vi "Reset all hightlights.vi"(8 "error in (no error)":errorcluster, 11 "Display State In in":T1={"logTable"=refnum, "max items"=500, "displaydata"=[], "data"=[], "Auto Scroll"=TRUE, "current item"=500, "col headers"=[], "Add to Top"=FALSE, "Auto resize"=TRUE, "col size"=[], "filters"=[], "color cells"=[]}) -> (0 "error out":errorcluster, 3 "Display State In out":T1={"logTable"=refnum, "max items"=500, "displaydata"=[], "data"=[], "Auto Scroll"=TRUE, "current item"=500, "col headers"=[], "Add to Top"=FALSE, "Auto resize"=TRUE, "col size"=[], "filters"=[], "color cells"=[]})   [LabVIEW 2013, in "UI-DisplayTable(dev).xctl"]
uses:
  UI-DisplayTable(dev).xctl
  State.ctl
  DEF-Filter.ctl
  <vilib>/Utility/miscctls.llb/LVRowAndColumnTypeDef.ctl
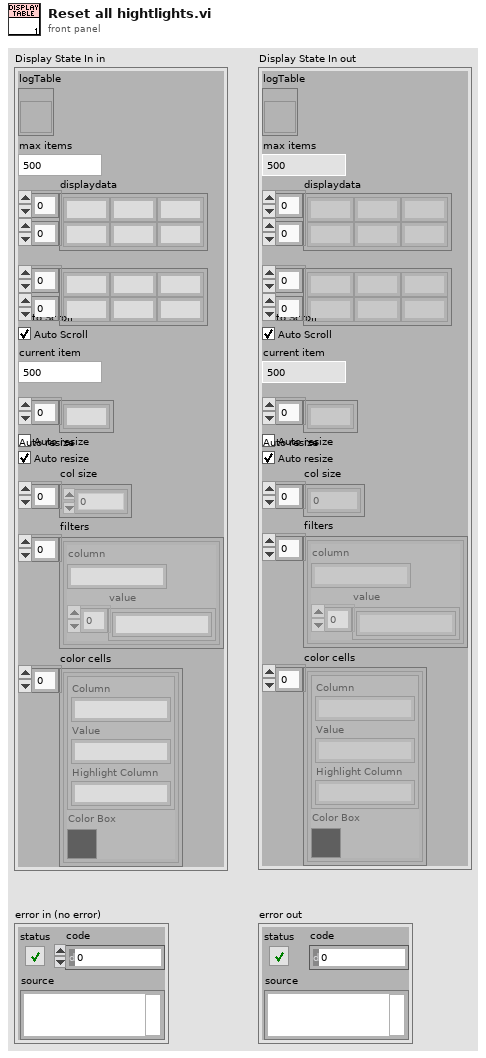
[diagram p1: front panel]
types:
  T1 = typedef "UI-DisplayTable(dev).xctl/State.ctl" = cluster{"logTable":refnum<vi>, "max items":i32, "displaydata":string[][], "data":string[][], "Auto Scroll":bool, "current item":i32, "col headers":string[], "Add to Top":bool, "Auto resize":bool, "col size":i32[], "filters":T2[], "color cells":cluster{"color cell":cluster{"Column":string, "Value":string, "Highlight Column":string}, "Color Box":u32}[]}
  T2 = typedef "UI-DisplayTable(dev).xctl/DEF-Filter.ctl" = cluster{"column":string, "value":string[]}
  T3 = typedef "LVRowAndColumnTypeDef.ctl" = cluster{"Row":i32, "Column":i32}
  T4 = cluster{"color cell":cluster{"Column":string, "Value":string, "Highlight Column":string}, "Color Box":u32}[]
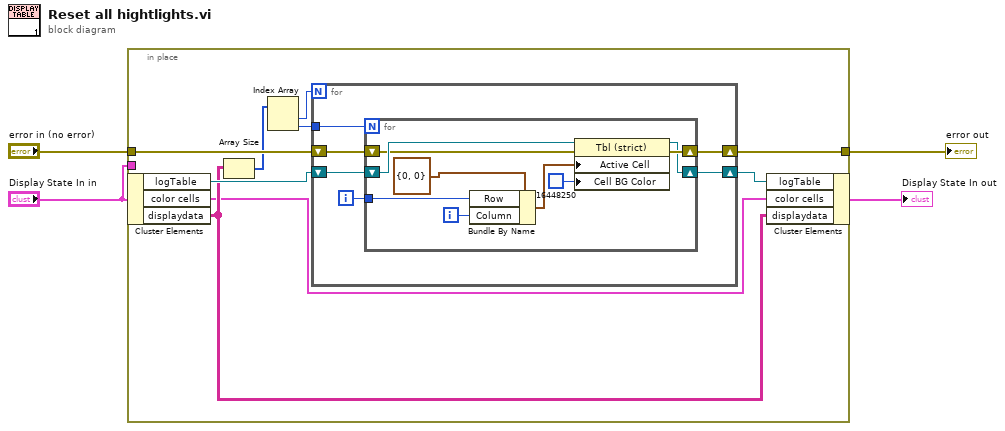
[diagram p0: block diagram]
diagram:
  n1 = in-place {
    in-place-border: "Display State In in" -> [_]
    in-place-border: "error in (no error)" -> [w13]
    in-place-border: [w12] -> w2
    n2 = in-place-cluster #1("Display State In in") -> ("logTable"=w11:refnum<vi>, "color cells"=w5:T4, "displaydata"=w9:string[][])
    n3 = Array Size(array=w9) -> (size(s)=w8:i32[])
    n4 = Index Array(array=w8) -> (element #1=w7:i32, element #2=w6:i32)  [unwired: 2 in]
    n5 = for {
      N: w7 -> [_]
      shift-right: [w17] -> w12
      shift-left: w13 -> [w18]
      shift-right: [w16] -> w10
      shift-left: w11 -> [w19]
      tunnel: w6 -> [w15]
      i -> [w14]
      n6 = for {
        N: w15 -> [_]
        shift-right: [w22] -> w16
        shift-left: w19 -> [w28]
        shift-right: [w25] -> w17
        shift-left: w18 -> [w26]
        tunnel: w14 -> [w21]
        i -> [w20]
        n7 = Bundle By Name(cluster=T3 {"Row"=0, "Column"=0} ("Active Cell:Active Cell"), "Row"=w21, "Column"=w20) -> (w23:T3)
        n8 = property class="Tbl (strict)"(reference=w28, error in=w26, "Active Cell"=w23, "Cell BG Color"=u32 16448250 ("Active Cell:Cell Background Color")) -> (reference out=w22:refnum<vi>, error out=w25:errorcluster)
      }
    }
    n9 = in-place-cluster #1("logTable"=w10, "color cells"=w5, "displaydata"=w9) -> (→"Display State In out":T1)
  }
  "error out" <- w2
